vi "ListBoxReference.vi"() -> ()   [LabVIEW 2020]
panel:
  in  "ListBox Ref":refnum<vi>
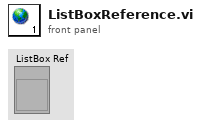
[diagram p1: front panel]
diagram:
